vi "Get Path.vi"(0 "Control ref":refnum<vi>, 11 "error in (no error)":errorcluster) -> (4 "Drona Path":string, 15 "error out":errorcluster)   [LabVIEW 2016, in "Drona basic.lvlib"]
uses:
  Drona basic.lvlib
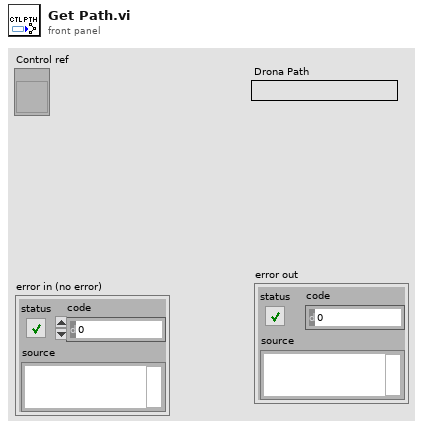
[diagram p1: front panel]
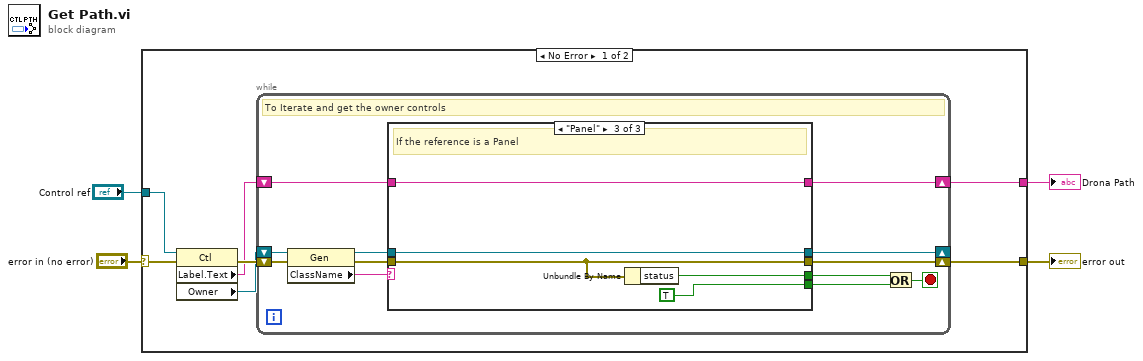
[diagram p0: block diagram]
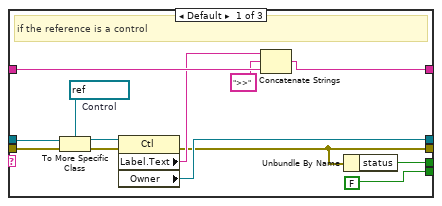
[diagram p2: hidden frame]
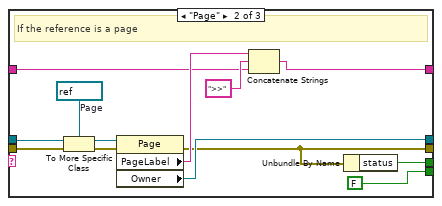
[diagram p3: hidden frame]
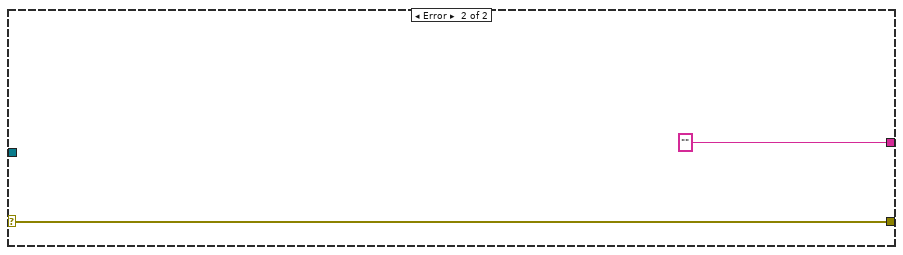
[diagram p4: hidden frame]
diagram:
  n1 = case shown="No Error" "error in (no error)" {
    selector: "error in (no error)" -> [w7 w56]
    tunnel: "Control ref" -> [w8 _]
    tunnel: [w6 w56] -> w2
    tunnel: [w5 "" ("Label.Text")] -> w1
    frame No Error {
      n2 = property class="Ctl"(reference=w8, error in=w7) -> (error out=w11:errorcluster, "Label.Text"=w9:string, "Owner"=w10:refnum<vi>)  [unwired: 1 out]
      n3 = while {
        shift-right: [w18] -> w6
        shift-left: w11 -> [w23]
        shift-right: [w16] -> w5
        shift-left: w9 -> [w17]
        shift-right: [w15] -> _
        shift-left: w10 -> [w22]
        stop <- w14 stop-if-true
        # "To Iterate and get the owner controls"
        n4 = property class="Gen"(reference=w22, error in=w23) -> (reference out=w20:refnum<vi>, error out=w19:errorcluster, "ClassName"=w21:string)
        n5 = case shown="\"Panel\"" w21 {
          tunnel: w20 -> [w34 w47 w52]
          tunnel: w19 -> [w36 w49 w51]
          tunnel: [w26 w39 w51] -> w18
          tunnel: [FALSE FALSE TRUE] -> w13
          tunnel: w17 -> [w30 w42 w53]
          tunnel: [w28 w41 w53] -> w16
          tunnel: [w31 w40 w52] -> w15
          tunnel: [w25 w38 w50] -> w12
          frame Default {
            w33 = refnum<vi> refnum  # Control
            # "if the reference is a control"
            n6 = To More Specific Class(target class=w33, reference=w34, error in=w36) -> (specific class reference=w32:refnum<vi>, error out=w35:errorcluster)
            n7 = property class="Ctl"(reference=w32, error in=w35) -> (error out=w26:errorcluster, "Label.Text"=w29:string, "Owner"=w31:refnum<vi>)  [unwired: 1 out]
            n8 = Concatenate Strings(w29, ">>" ("string"), w30) -> (w28:string)
            n9 = Unbundle By Name(w26) -> ("status"=w25:bool)
          }
          frame "Page" {
            w46 = refnum<vi> refnum  # Page
            # "If the reference is a page"
            n10 = To More Specific Class(target class=w46, reference=w47, error in=w49) -> (specific class reference=w45:refnum<vi>, error out=w48:errorcluster)
            n11 = property class="Page"(reference=w45, error in=w48) -> (error out=w39:errorcluster, "PageLabel"=w43:string, "Owner"=w40:refnum<vi>)  [unwired: 1 out]
            n12 = Concatenate Strings(w43, ">>" ("string"), w42) -> (w41:string)
            n13 = Unbundle By Name(w39) -> ("status"=w38:bool)
          }
          frame "Panel" {
            # "If the reference is a Panel"
            n14 = Unbundle By Name(w51) -> ("status"=w50:bool)
          }
        }
        n15 = Or(x=w12, y=w13) -> (x .or. y?=w14:bool)
      }
    }
    frame Error {
    }
  }
  "error out" <- w2
  "Drona Path" <- w1
